vi "Sequence State Change Event Callback.vi"(4 "Sequence State Change Event Data":refnum<user-event>, 5 "Event Data":cluster{"sender":refnum<k24>, "e":refnum<k24>}, 6 "Control Ref":refnum<k24>, 7 "Event Common Data":T1) -> ()   [LabVIEW 2020, in "NI_VS Sequence Execution Interface.lvlib"]
uses:
  <vilib>/NI VeriStand/Execution/SequenceExecutionInterface/NI_VS Sequence Execution Interface.lvlib
  NationalInstruments.VeriStand.ClientAPI
  <vilib>/NI VeriStand/Execution/SequenceExecutionInterface/Sequence State Change Event Data.ctl
  <vilib>/NI VeriStand/Execution/SequenceExecutionInterface/Sequence Execution State.ctl
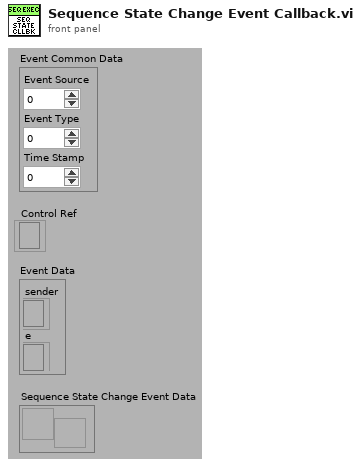
[diagram p1: front panel]
types:
  T1 = cluster{"Event Source":i32, "Event Type":u32, "Time Stamp":u32}
  T2 = typedef "NI_VS Sequence Execution Interface.lvlib/Sequence State Change Event Data.ctl" = cluster{"Sequence Name":string, "State":T3, "Aborted":bool}
  T3 = typedef "NI_VS Sequence Execution Interface.lvlib/Sequence Execution State.ctl" = enum16{"Idle", "Running", "SingleStepping", "Paused", "Stopped"}
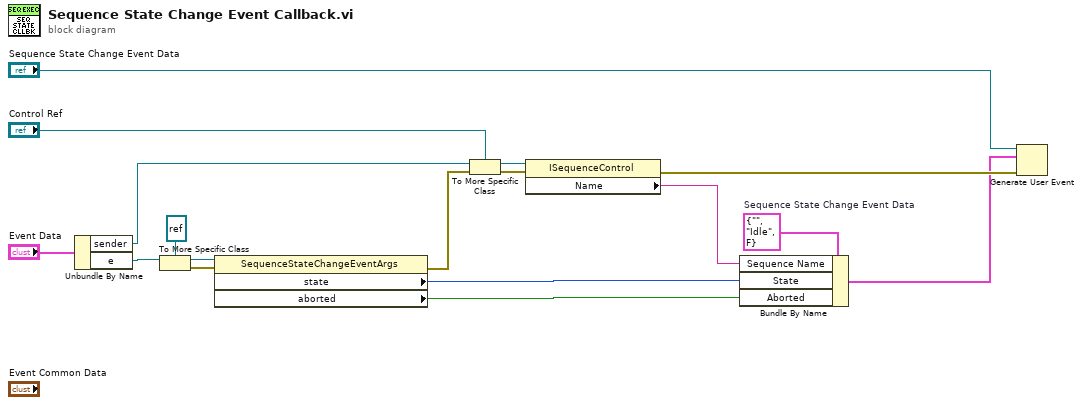
[diagram p0: block diagram]
diagram:
  w1 = T2 {"Sequence Name"="", "State"=enum."Idle", "Aborted"=FALSE}  # Sequence State Change Event Data
  n1 = Unbundle By Name("Event Data") -> ("sender"=w15:refnum<k24>, "e"=w12:refnum<k24>)
  n2 = To More Specific Class(target class=refnum<k24> refnum, reference=w12) -> (specific class reference=w10:refnum<k24>, error out=w9:errorcluster)  [unwired: 1 in]
  n3 = property class="SequenceStateChangeEventArgs"(reference=w10, error in=w9) -> (error out=w8:errorcluster, "state"=w5:i32, "aborted"=w4:bool)  [unwired: 1 out]
  n4 = To More Specific Class(target class="Control Ref", reference=w15, error in=w8) -> (specific class reference=w13:refnum<k24>, error out=w7:errorcluster)
  n5 = property class="ISequenceControl"(reference=w13, error in=w7) -> (error out=w17:errorcluster, "Name"=w6:string)  [unwired: 1 out]
  n6 = Bundle By Name(cluster=w1, "Sequence Name"=w6, "State"=w5, "Aborted"=w4) -> (w2:T2)
  n7 = Generate User Event(user event="Sequence State Change Event Data", event data cluster=w2, error in=w17) -> ()  [unwired: 1 in, 2 out]
